vi "GDS_MO_GetEnergy180311.vi"() -> (9 "AEnergy":dbl=5.0)   [LabVIEW 2015]
uses:
  C/Program Files/National Instruments/LabVIEW 2015/user.lib/caLab/Private/Get_PV-1D.vi
panel:
  out "SPEC:mono132":dbl
  out "SPEC:INC":dbl
  out "retrunvalue":i32
  out "SPEC:BUSY":dbl
  # "GetEnergy"
  # "EPICS"
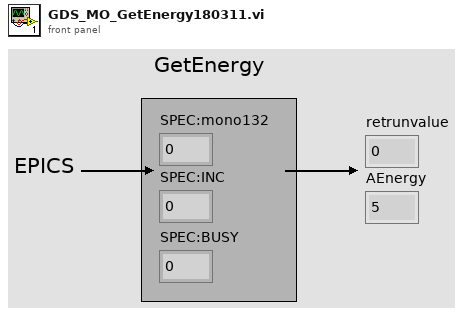
[diagram p1: front panel]
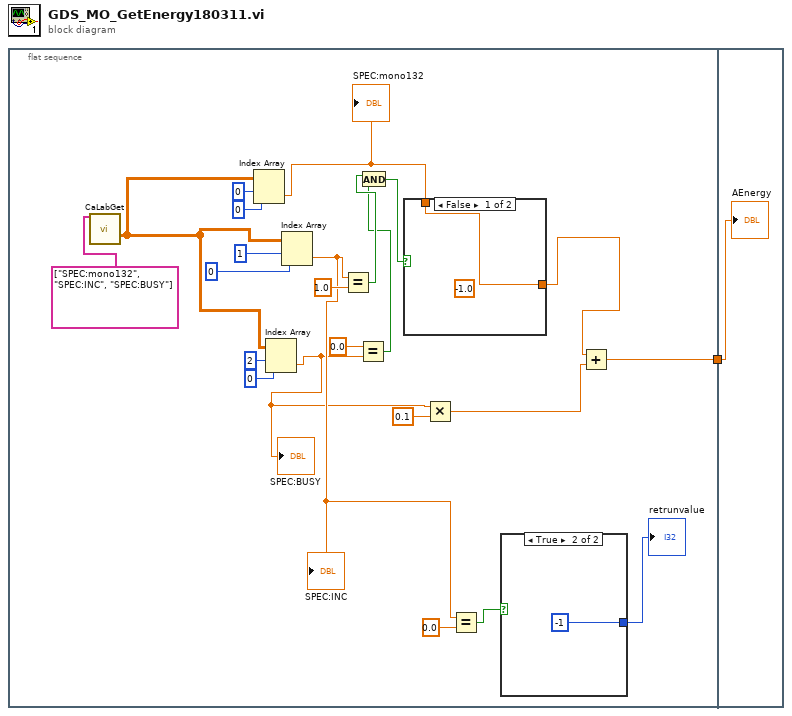
[diagram p0: block diagram]
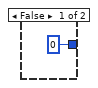
[diagram p2: hidden frame]
diagram:
  n1 = flat-sequence {
    tunnel: [w2] -> w1
    tunnel: w1 -> [w29]
    frame #0 {
      n2 = call-poly "CaLabGet.vi"("PV Names"=string[] ["SPEC:mono132", "SPEC:INC", "SPEC:BUSY"]) -> ("Value Array (number)"=w11:dbl[][])  [unwired: 8 in, 6 out]
      n3 = Index Array(array=w11, index (row)=0, index (col)=0 ("disabled index (col)")) -> (element=w12:dbl)
      "SPEC:mono132" <- w12
      n4 = Index Array(array=w11, index (row)=2, index (col)=0 ("disabled index (col)")) -> (element=w6:dbl)
      "SPEC:BUSY" <- w6
      n5 = Index Array(array=w11, index (row)=1, index (col)=0 ("disabled index (col)")) -> (element=w10:dbl)
      "SPEC:INC" <- w10
      n6 = Equal?(x=w10, y=1.0) -> (x = y?=w15:bool)
      n7 = Equal?(x=0.0, y=w6) -> (x = y?=w14:bool)
      n8 = And(x=w15, y=w14) -> (x .and. y?=w13:bool)
      n9 = case shown="False" w13 {
        tunnel: [w27 w28] -> w4
        tunnel: w12 -> [w27 w28]
        frame False {
          (unwired) -1.0
        }
        frame True {
        }
      }
      n10 = Multiply(x=w6, y=0.1) -> (x*y=w3:dbl)
      n11 = Equal?(x=w10, y=0.0) -> (x = y?=w8:bool)
      n12 = case shown="True" w8 {
        tunnel: [0 -1] -> w7
        frame False {
        }
        frame True {
        }
      }
      "retrunvalue" <- w7
      n13 = Add(x=w4, y=w3) -> (x+y=w2:dbl)
    }
    frame #1 {
      "AEnergy" <- w29
    }
  }
